vi "Configure Power On State.vi"(8 "error in (no error)":errorcluster, 10 "Memory Location (0: Default Location)":i32(ring) items=["Default Location", "Memory Location 0", "Memory Location 1", "Memory Location 2", "Memory Location 3", "Memory Location 4", "Memory Location 5", "Memory Location 6", "Memory Location 7", "Memory Location 8", "Memory Location 9"], 11 "VISA resource name":refnum<visa-resource-name>) -> (0 "error out":errorcluster, 3 "VISA resource name out":refnum<visa-resource-name>)   [LabVIEW 2020, in "Keysight E36300 Series.lvlib"]
doc: "Specifies whether the power supply's power-on state is the default state or the state stored in one of ten memory locations."
uses:
  Keysight E36300 Series.lvlib
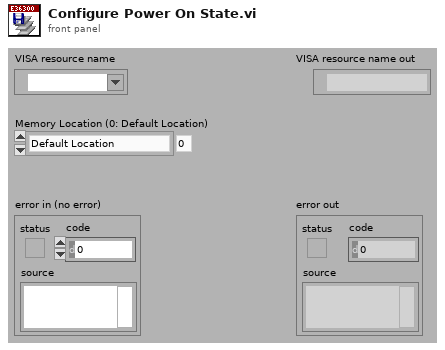
[diagram p1: front panel]
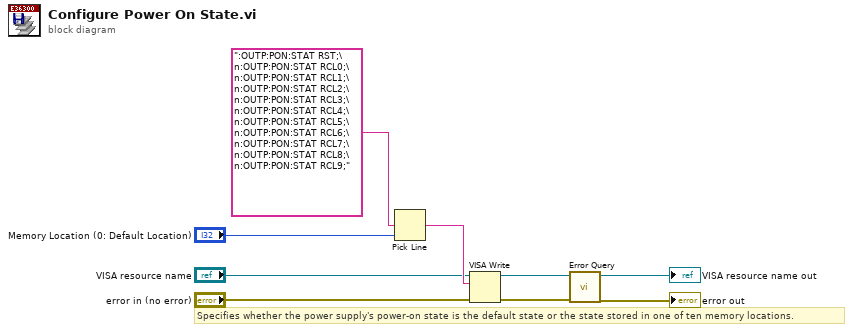
[diagram p0: block diagram]
diagram:
  # "Specifies whether the power supply's power-on state is the default state or the state stored in one of ten memory locations."
  n1 = Pick Line(multi-line string=":OUTP:PON:STAT RST;\n:OUTP:PON:STAT RCL0;\n:OUTP:PON:STAT RCL1;\n:OUTP:PON:STAT RCL2;\n:OUTP:PON:STAT RCL3;\n:OUTP:PON:STAT RCL4;\n:OUTP:PON:STAT RCL5;\n:OUTP:PON:STAT RCL6;\n:OUTP:PON:STAT RCL7;\n:OUTP:PON:STAT RCL8;\n:OUTP:PON:STAT RCL9;", line index="Memory Location (0: Default Location)") -> (output string=w7:string)  [unwired: 1 in]
  n2 = VISA Write(VISA resource name="VISA resource name", write buffer=w7, error in (no error)="error in (no error)") -> (VISA resource name out=w4:refnum<visa-resource-name>, error out=w3:errorcluster)  [unwired: 1 out]
  n3 = call "Error Query.vi"("error in (no error)"=w3, "VISA resource name"=w4) -> ("error out"=→"error out":errorcluster, "VISA resource name out"=→"VISA resource name out":refnum<visa-resource-name>)  [unwired: 6 in, 2 out]
